vi "ep_Check Trigger and Time.vi"(7 "trigger? (F)":bool, 8 "error in (no error)":errorcluster, 10 "triggers per cycle":u8=2, 11 "trigger/positions [s]":dbl[](array[numeric])) -> (0 "error out":errorcluster, 2 "dup triggers per cycle":u8, 3 "dup trigger/positions [s]":dbl[](array[numeric]))   [LabVIEW 2013, in "NI_EP_Power Measurement.lvlib"]
uses:
  <vilib>/addons/Electrical Power/Power Measurement/NI_EP_Power Measurement.lvlib
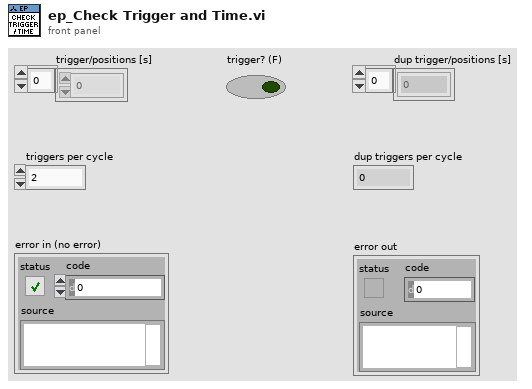
[diagram p1: front panel]
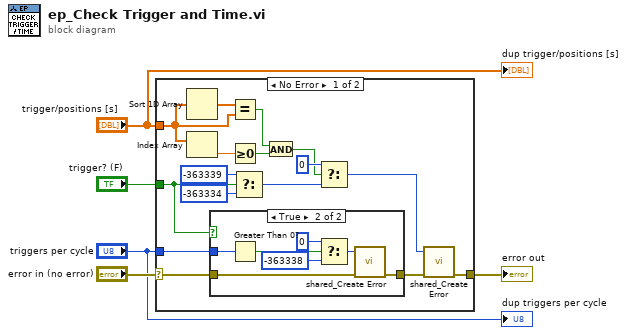
[diagram p0: block diagram]
diagram:
  n1 = case shown="No Error" "error in (no error)" {
    selector: "error in (no error)" -> [w21 w30]
    tunnel: [w13 w30] -> w4
    tunnel: "trigger/positions [s]" -> [w15 _]
    tunnel: "triggers per cycle" -> [w14 _]
    tunnel: "trigger? (F)" -> [w6 _]
    frame No Error {
      n2 = Sort 1D Array(array=w15) -> (sorted array=w20:dbl[])
      n3 = Index Array(array=w15) -> (element=w16:dbl)  [unwired: 1 in]
      n4 = case shown="True" w6 {
        tunnel: w21 -> [w22 w29]
        tunnel: [w22 w25] -> w18
        tunnel: w14 -> [_ w23]
        frame False {
        }
        frame True {
          n5 = Greater Than 0?(x=w23) -> (x > 0?=w26:bool)
          n6 = Select(t=0 ("error code (0)"), s=w26, f=-363338 ("error code (0)")) -> (s? t:f=w24:i32)
          n7 = call <vilib>:"shared_Create Error.vi"("error in (no error)"=w29, "error code (0)"=w24) -> ("error out"=w25:errorcluster)  [unwired: 9 in]
        }
      }
      n8 = Equal?(x=w20, y=w15) -> (x = y?=w8:bool)
      n9 = Greater Or Equal To 0?(x=w16) -> (x >= 0?=w9:bool)
      n10 = Select(t=-363339 ("error code (0)"), s=w6, f=-363334 ("error code (0)")) -> (s? t:f=w10:i32)
      n11 = And(x=w8, y=w9) -> (x .and. y?=w7:bool)
      n12 = Select(t=0 ("error code (0)"), s=w7, f=w10) -> (s? t:f=w17:i32)
      n13 = call <vilib>:"shared_Create Error.vi"("error in (no error)"=w18, "error code (0)"=w17) -> ("error out"=w13:errorcluster)  [unwired: 9 in]
    }
    frame Error {
    }
  }
  "error out" <- w4
  "dup triggers per cycle" <- "triggers per cycle"
  "dup trigger/positions [s]" <- "trigger/positions [s]"
